vi "Test_API_RunLoggerStopLoggerGetStatus_ValidStatus.vi"(8 "error in (no error)":errorcluster, 11 "TestCase in":refnum<class "TestLocalLogInstance.lvclass">) -> (0 "error out":errorcluster, 3 "TestCase out":refnum<class "TestLocalLogInstance.lvclass">)   [LabVIEW 2017, in "TestLocalLogInstance.lvclass"]
uses:
  TestLocalLogInstance.lvclass
  Source/Composed Log/LoggerReference/LoggerReference.lvclass/LoggerReference.ctl
  9a0b009a-159a-478b-8bd0-efcaa49947a6.vi
  Source/Composed Log/LoggerReference/Return Aggregate Queues.vi
  Source/Composed Log/LoggerReference/Add Aggregate Log.vi
  9a0b009a-159a-478b-8bd0-efcaa49947a6.vi/c8a11b63-a48b-4926-811c-e01bafe01fc4.vi
  Source/Composed Log/LoggerReference/Send Add Sink.vi
  Source/LVQueue Sink/LVQueue Sink.lvclass
  C:/CS/Internal/LabVIEW/Logger/Source/Composed Log/Log Sink/Log Sink.lvclass
  Source/Composed Log/Application Logger/Launch Worker Loop.vi
  Source/Composed Log/LoggerReference/Initialize Logger Instance.vi
  Source/Composed Log/LoggerReference/LoggerReference.lvclass
  Source/Composed Log/IErrorFormat/IErrorFormat.lvclass
  Source/Composed Log/Log Sink/Log Sink.lvclass
  <vilib>/addons/_JKI Toolkits/VI Tester/TestCase.llb/TestCase.lvclass
  C:/Program Files (x86)/National Instruments/LabVIEW 2017/vi.lib/addons/_JKI Toolkits/VI Tester/TestCase.llb/TestCase.lvclass
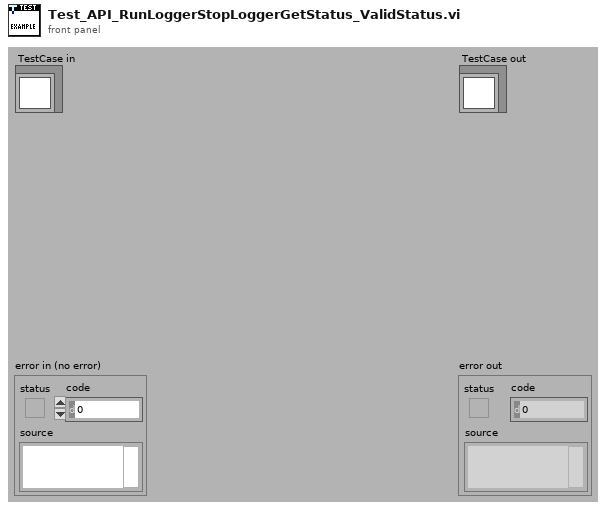
[diagram p1: front panel]
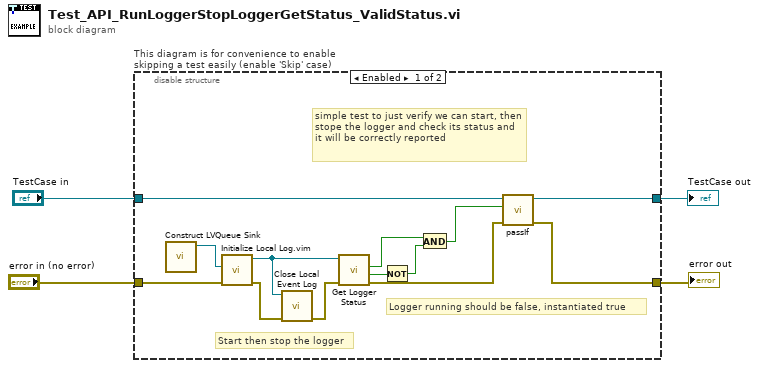
[diagram p0: block diagram]
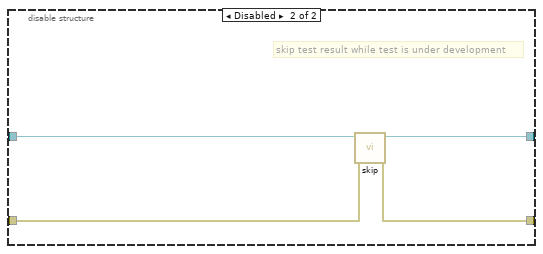
[diagram p2: hidden frame]
diagram:
  n1 = disable-structure "This diagram is for convenience to enable skipping a test easily (enable 'Skip' case)" shown="Enabled" {
    disable-tunnel: "TestCase in" -> [w16 w21]
    disable-tunnel: [w17 w19] -> w1
    disable-tunnel: [w15 w20] -> w3
    disable-tunnel: "error in (no error)" -> [w14 w18]
    frame Enabled {
      # "Logger running should be false, instantiated true"
      # "Start then stop the logger"
      # "simple test to just verify we can start, then stope the logger and check its status and it will be correctly reported"
      n2 = call "Construct LVQueue Sink.vi"() -> ("LVQueue Sink out"=w13:refnum<class "LVQueue Sink.lvclass">)  [unwired: 10 in, 1 out]
      n3 = call "Initialize Local Log.vim"("error in (no error)"=w14, "Startup Sink(s)"=w13) -> ("error out"=w9:errorcluster, "Log Instance Reference"=w8:refnum<class "LoggerReference.lvclass">)  [unwired: 7 in, 1 out]
      n4 = call "Close Local Event Log.vi"("error in (no error)"=w9, "Log Instance"=w8) -> ("error out"=w7:errorcluster)  [unwired: 9 in]
      n5 = call "Get Logger Status.vi"("error in (no error)"=w7, "LoggerReference in"=w8) -> ("error out"=w6:errorcluster, "Logger Running?"=w12:bool, "Logger Instantiated?"=w11:bool)  [unwired: 6 in, 1 out]
      n6 = Not(x=w12) -> (.not. x?=w5:bool)
      n7 = And(x=w11, y=w5) -> (x .and. y?=w10:bool)
      n8 = call-dynamic "passIf.vi"("error in (no error)"=w6, "pass"=w10, "TestCase in"=w16) -> ("error out"=w15:errorcluster, "TestCase out"=w17:refnum<class "TestLocalLogInstance.lvclass">)  [unwired: 7 in]
    }
    frame Disabled {
      # "skip test result while test is under development"
      n9 = call <vilib>:"skip.vi"("error in (no error)"=w18, "TestCase in"=w21) -> ("error out"=w20:errorcluster, "TestCase out"=w19:refnum<class "TestLocalLogInstance.lvclass">)  [unwired: 8 in]
    }
  }
  "error out" <- w3
  "TestCase out" <- w1
